vi "Update Monitor State.vi"(8 "error in (no error)":errorcluster, 10 "Monitor Running":bool, 11 "LabActor in":refnum<class "LabActor.lvclass">) -> (0 "error out":errorcluster, 3 "LabActor out":refnum<class "LabActor.lvclass">)   [LabVIEW 2021, in "LabActor.lvclass"]
uses:
  LabActor.lvclass
  C:/GitHub/LabActor/Template Module/Template Module.lvclass
  C:/Program Files/National Instruments/LabVIEW 2021/vi.lib/ActorFramework/Actor/Actor.lvclass
  NHMFL_Core/Libraries/Instruments/Results/File Path Result/File Path Result.lvclass
  C:/GitHub/NHMFL_Core/Libraries/Instruments/Results/Acquired Result/Acquired Result.lvclass
  C:/GitHub/LabActor/Publish-Subscribe/Interfaces/Information/Information.lvclass
  Publish-Subscribe/Context.ctl
  Template Module/Template Module.lvclass/Template Module.ctl
  <vilib>/ActorFramework/Actor/Actor.lvclass/Actor.ctl
  <vilib>/ActorFramework/Message Enqueuer/Message Enqueuer.lvclass/Message Enqueuer.ctl
  NHMFL_Core/Libraries/Instruments/Results/Acquired Result/Acquired Result.lvclass/Acquired Result.ctl
  Publish-Subscribe/Interfaces/Subscriber Messages/Information Msg/Information Msg.lvclass/Information Msg.ctl
  Template Module/Read Name.vi
  NHMFL_Core/Libraries/Instruments/Results/Acquired Result/Write Sender.vi
  <vilib>/ActorFramework/Message Enqueuer/Init from Existing Queue.vi
  <vilib>/ActorFramework/Message Enqueuer/Enqueue.vi
  Publish-Subscribe/Interfaces/Subscriber Messages/Information Msg/Information Msg.lvclass
  C:/Program Files/National Instruments/LabVIEW 2021/vi.lib/ActorFramework/Message/Message.lvclass
  <vilib>/ActorFramework/Message Priority Queue/Priority Enqueue.vi
  Controllers/Application Controller/Application Controller.lvclass
  <vilib>/ActorFramework/Message Enqueuer/Message Enqueuer.lvclass
  <vilib>/ActorFramework/Actor/Actor.lvclass
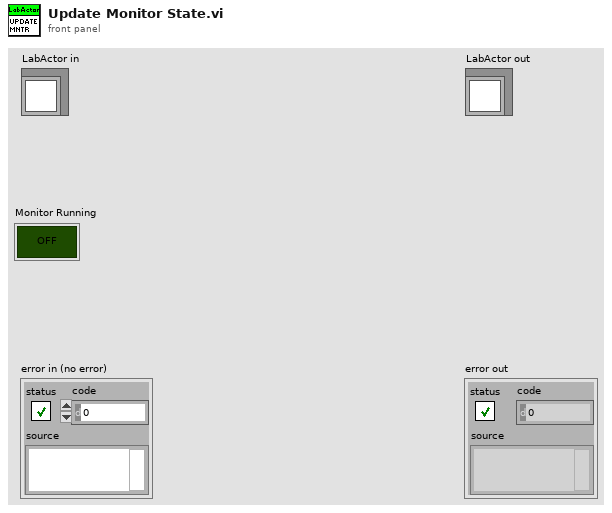
[diagram p1: front panel]
types:
  T1 = typedef "Context.ctl" = cluster{"Topic":string, "Source":string}
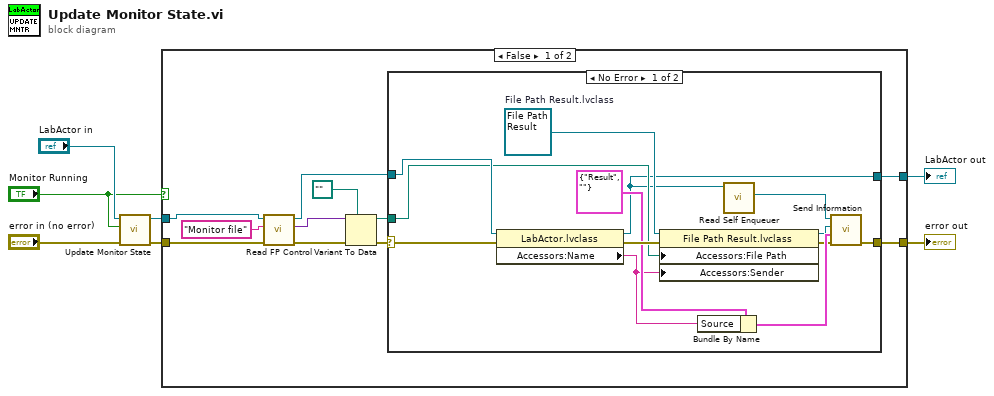
[diagram p0: block diagram]
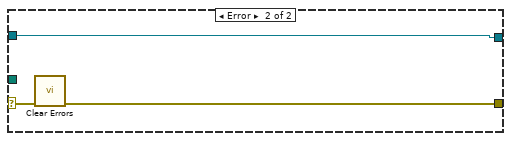
[diagram p2: hidden frame]
diagram:
  n1 = call-parent "Update Monitor State.vi"("error in (no error)"="error in (no error)", "Monitor Running"="Monitor Running", "Application Controller in"="LabActor in") -> ("error out"=w4:errorcluster, "Application Controller out"=w5:refnum<class "LabActor.lvclass">)  [unwired: 7 in]
  n2 = case shown="False" "Monitor Running" {
    tunnel: w5 -> [w18 w35]
    tunnel: w4 -> [w11 w36]
    tunnel: [w9 w36] -> w2
    tunnel: [w8 w35] -> w1
    frame False {
      n3 = call-dynamic "Read FP Control.vi"("error in (no error)"=w11, "Control Name"="Monitor file", "Measure Object in"=w18) -> ("error out"=w15:errorcluster, "Control Value"=w12:variant, "Measure Object out"=w17:refnum<class "LabActor.lvclass">)  [unwired: 5 in, 1 out]
      n4 = Variant To Data(error in=w15, type=path "", Variant=w12) -> (data=w13:path, error out=w10:errorcluster)
      n5 = case shown="No Error" w10 {
        selector: w10 -> [w27 w33]
        tunnel: w17 -> [w29 w34]
        tunnel: w13 -> [w28 _]
        tunnel: [w20 w32] -> w9
        tunnel: [w23 w34] -> w8
        frame No Error {
          w31 = refnum<class "File Path Result.lvclass"> refnum  # File Path Result.lvclass
          n6 = property class="LabActor.lvclass"(reference=w29, error in=w27) -> (reference out=w23:refnum<class "LabActor.lvclass">, error out=w30:errorcluster, "Accessors:Name"=w19:string)
          n7 = property class="File Path Result.lvclass"(reference=w31, error in=w30, "Accessors:File Path"=w28, "Accessors:Sender"=w19) -> (reference out=w22:refnum<class "File Path Result.lvclass">, error out=w21:errorcluster)
          n8 = Bundle By Name(cluster=T1 {"Topic"="Result", "Source"=""} ("Context"), "Source"=w19) -> (w26:T1)
          n9 = call <vilib>:"Read Self Enqueuer.vi"("Actor"=w23) -> ("Self Enqueuer"=w24:refnum<class "Message Enqueuer.lvclass">)  [unwired: 10 in]
          n10 = call "Send Information.vi"("error in (no error)"=w21, "Context"=w26, "Information"=w22, "Message Enqueuer"=w24) -> ("error out"=w20:errorcluster)  [unwired: 6 in, 1 out]
        }
        frame Error {
          n11 = call <vilib>:"Clear Errors.vi"("error in (no error)"=w33) -> ("error out"=w32:errorcluster)  [unwired: 5 in, 1 out]
        }
      }
    }
    frame True {
    }
  }
  "error out" <- w2
  "LabActor out" <- w1
